vi "Fpga-Uart-State-Machine.vi"(6 "TX FIFO In":refnum<k21>="HT-UART_TX", 7 "RXD Pin In":refnum<k21>="UserRTL_d_microblaze_wrapper\\uart_rtl_rxd", 8 "RX FIFO In":refnum<k21>="TH-UART_RX", 9 "TXD Pin In":refnum<k21>="UserRTL_d_microblaze_wrapper\\uart_rtl_txd", 10 "Baud Rate":u32(ring)=128000 items=["110"=110, "300"=300, "1200"=1200, "2400"=2400, "4800"=4800, "9600"=9600, "19200"=19200, "38400"=38400, "57600"=57600, "115200"=115200, "128000"=128000, "230400"=230400, "460800"=460800, "921600"=921600], 11 "FPGA Clock Rate (MHz)":u32=100) -> ()   [LabVIEW 2018]
uses:
  <vilib>/Platform/TimedLoop/XDataNode/timing_clust.ctl
  <vilib>/Platform/TimedLoop/XDataNode/nitl_modes.ctl
  <vilib>/Platform/TimedLoop/XDataNode/wakeup.ctl
  UART.RX.States.2.ctl
  UART.RX.States.ctl
  <vilib>/rvi/Emulation/niFpgaSctlEmulationGetInTimedLoop.vi
  <vilib>/rvi/Emulation/niFpgaEmulationReportErrorSimple.vi
  <vilib>/rvi/Emulation/niFpgaGetClockAttributes.vi
  <vilib>/rvi/Emulation/niFpgaCriticalErrorInLSC.vi
  <vilib>/rvi/eio/common/nirviEmuTemplateMethod_errors.vi
  <vilib>/rvi/DataTransferAndStorage/Container/Common/niFpgaContainerExecOnDevCompGetState.vi
  <vilib>/rvi/Emulation/niFpgaEmulationIsFPGAContextNoSignature.vi
  <vilib>/rvi/errors/niFpgaSetErrorForExecOnDevCompSimple.vi
  <vilib>/rvi/eio/common/nirviEmuReportErrorAndStop.vi
  <vilib>/rvi/DataTransferAndStorage/Container/Common/niFpgaContainerGetUniqueNameForEmu.vi
  <vilib>/rvi/FIFO/Fifo_Resource/nirvififoEmulationSetSize.vi
  <vilib>/rvi/FIFO/Fifo_Resource/nirviFifoEmulationQueueMgr.vi
  <instcachedir>/0/nirviFifoEmulationQueueMgr_E5CAEC123FF24DC58D834DCA3CDAA9B5.lvgen/nirviFifoEmulationQueueMgr_E5CAEC123FF24DC58D834DCA3CDAA9B5_001.vi
  <vilib>/rvi/FIFO/Fifo_Resource/nirvififoEmulationDetermineInputValidOut.vi
  <vilib>/rvi/FIFO/Fifo_Resource/nirvififoEmulationCreateLock.vi
  <vilib>/rvi/Emulation/niFpgaProcessEmulError.vi
  <vilib>/rvi/FIFO/Fifo_Resource/nirvififoEmulationObtainLock.vi
  <vilib>/rvi/FIFO/Fifo_Resource/nirvififoEmulationReleaseLock.vi
  <vilib>/rvi/occurrence/nirviWaitOnOccurrenceBase.vi
  <vilib>/rvi/errors/nirviReportUnexpectedCaseInternalError.vi
  <vilib>/rvi/errors/nirviReportUnexpectedCaseInternalError (U32).vi
  <vilib>/Utility/error.llb/Clear Errors.vi
  <vilib>/rvi/interface/RandomDataEmulation/niFpgaRandomDataHandleErrors.vi
  <vilib>/Platform/TimedLoop/XDataNode/XDataNode.xnode
  <vilib>/eio/EIONode/EIONode.xnode
  <vilib>/rvi/DataTransferAndStorage/Container/XNode/niFpgaContainer.xnode
  <vilib>/rvi/FIFO/Fifo_Resource/niFpgaFifoEmulationRefIn.vi
  <vilib>/Platform/TimedLoop/XDataNode/XDNodeRunTimeDep.lvlib
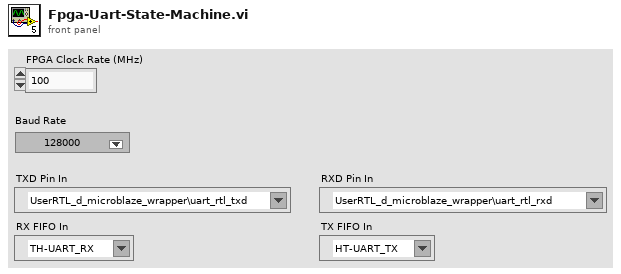
[diagram p1: front panel]
types:
  T1 = typedef "XDNodeRunTimeDep.lvlib/timing_clust.ctl" = cluster{"Expected End [f-1]":u64, "Actual End [f-1]":u64, "Finished Late? [f-1]":bool, "Expected End [i-1]":u64, "Actual End [i-1]":u64, "Finished Late? [i-1]":bool, "Expected Start [i]":u64, "Actual Start [i]":u64, "Expected Start [f]":u64, "Actual Start [f]":u64, "Source Name":string, "Structure Name":string, "Period":i64, "Deadline":i64, "Offset":i64, "Start":i64, "Priority":i32, "Timeout":i32, "Mode":T2, "Wakeup Reason":T3, "Error":errorcluster, "Source Type":string, "Secondary Source Type":string, "Global End Time":u64, "Global Start Time":u64, "Frame Duration":u64, "Iteration Duration":u64, "Assigned CPU":i32, "I/O Scan Engine Mode":u32}
  T2 = typedef "XDNodeRunTimeDep.lvlib/nitl_modes.ctl" = enum32{"No Change", "Process missed periods, maintain original phase", "Discard missed periods, maintain original phase", "Process missed periods, ignore original phase", "Discard missed periods, ignore original phase"}
  T3 = typedef "XDNodeRunTimeDep.lvlib/wakeup.ctl" = enum32{"Normal", "Aborted", "Asynchronous wakeup", "Timing source error", "Timed loop error", "Timeout"}
  T4 = typedef "UART.RX.States.2.ctl" = enum16{"No-Wait", "Wait-Half", "Wait-Full", "Wait-One-and-a-Half"}
  T5 = typedef "UART.RX.States.ctl" = enum16{"Read-StartBit", "Read-DataBits", "Read-Parity", "Read-StopBit", "Shift"}
  T6 = enum16{"Wait.for.New", "Send.StartBit", "Send.DataBits", "Send.Parity", "Send.StopBit"}
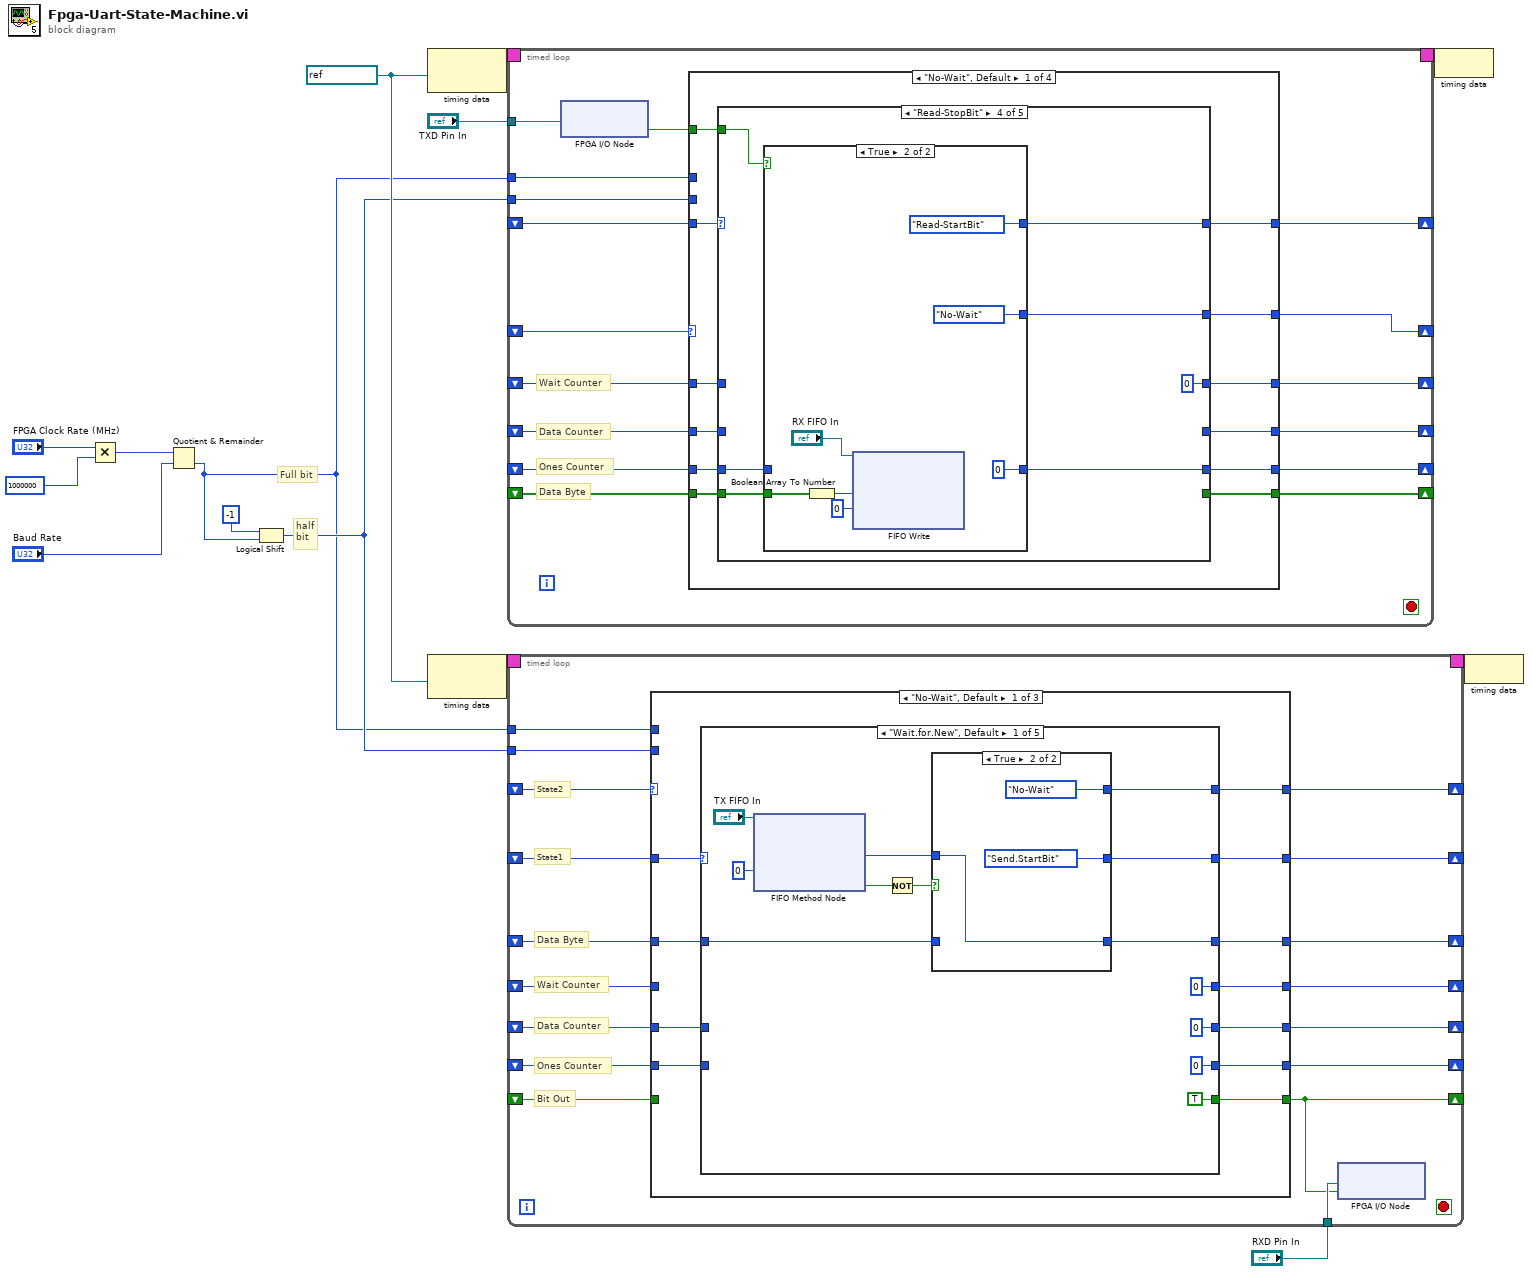
[diagram p0: block diagram]
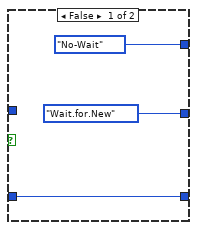
[diagram p2: hidden frame]
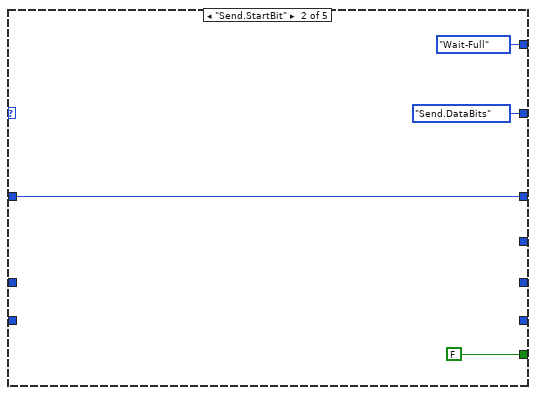
[diagram p3: hidden frame]
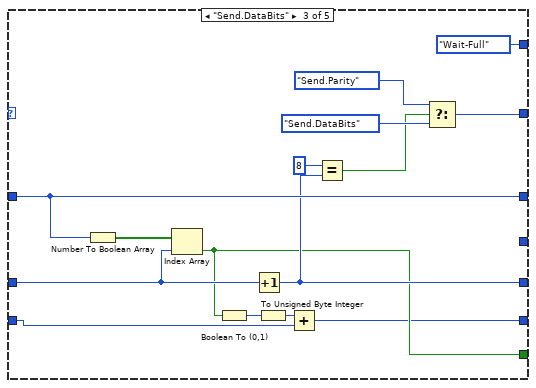
[diagram p4: hidden frame]
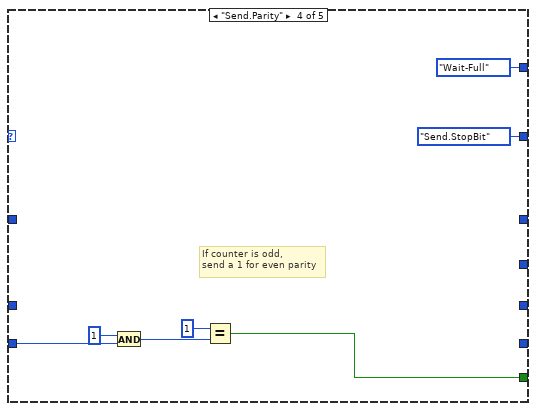
[diagram p5: hidden frame]
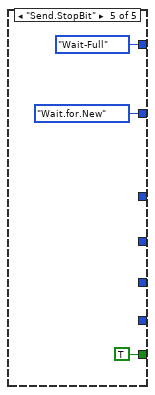
[diagram p6: hidden frame]
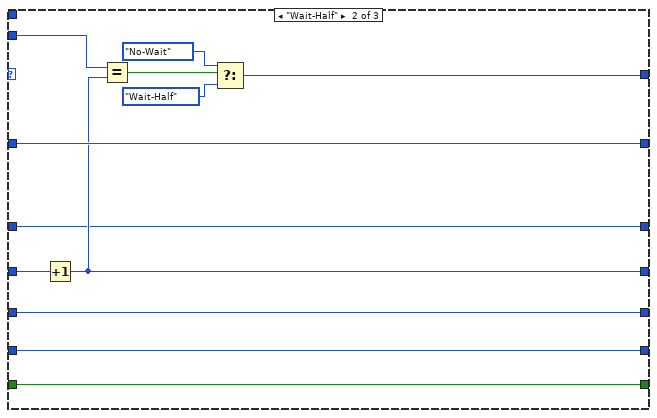
[diagram p7: hidden frame]
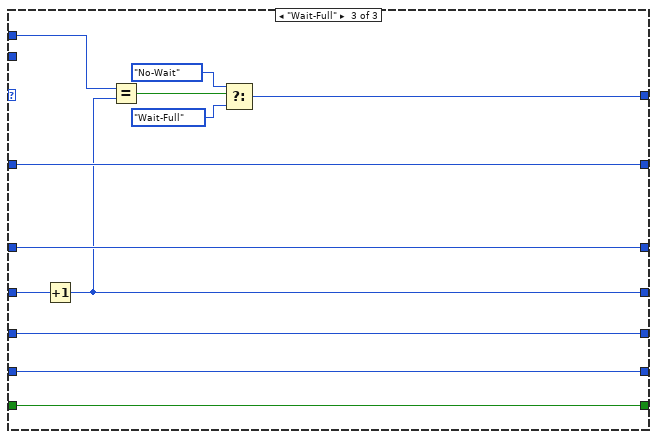
[diagram p8: hidden frame]
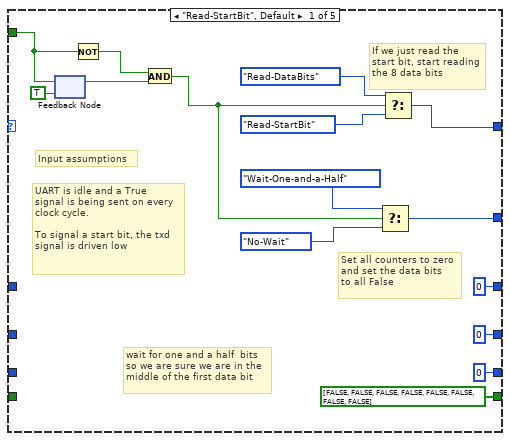
[diagram p9: hidden frame]
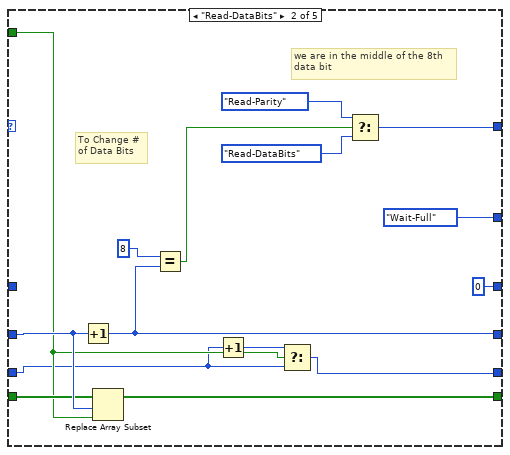
[diagram p10: hidden frame]
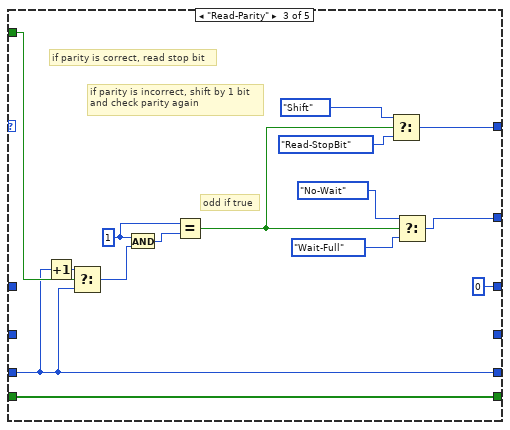
[diagram p11: hidden frame]
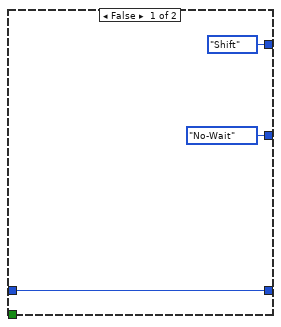
[diagram p12: hidden frame]
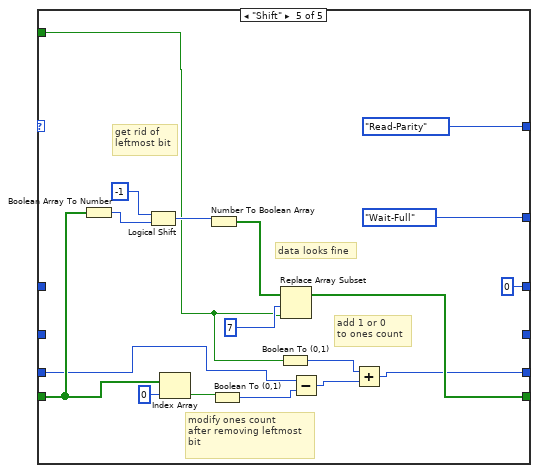
[diagram p13: hidden frame]
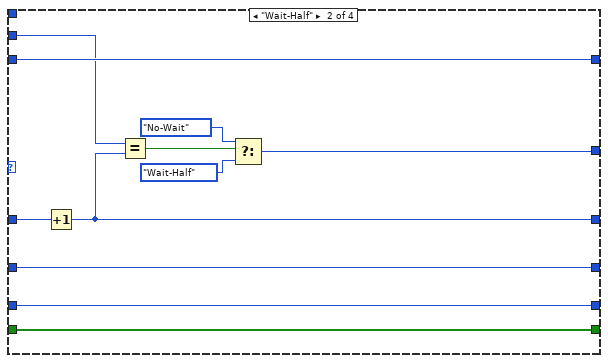
[diagram p14: hidden frame]
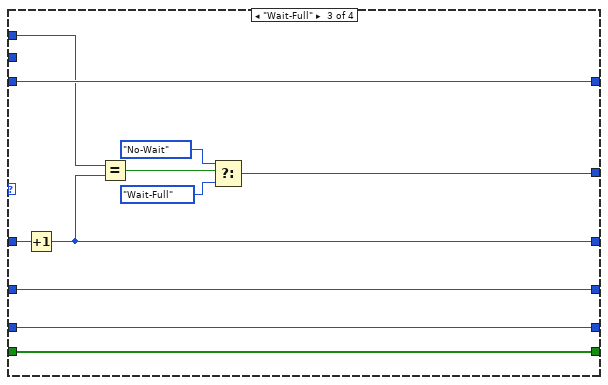
[diagram p15: hidden frame]
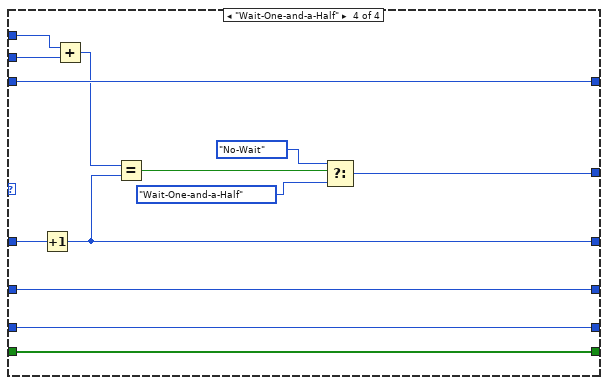
[diagram p16: hidden frame]
diagram:
  w3 = refnum<k21> "100MHz" ("Source Name")
  # "half\nbit"
  # "Full bit"
  n1 = Multiply(x="FPGA Clock Rate (MHz)", y=u32 1000000) -> (x*y=w13:u32)
  n2 = Quotient & Remainder(x=w13, y="Baud Rate") -> (floor(x/y)=w1:u32)  [unwired: 1 out]
  n3 = Logical Shift(y=i16 -1, x=w1) -> (x << y=w2:u32)
  n4 = node-c288(w3) -> (w10:T1)
  n5 = node-c288(w3) -> (w6:T1)
  n6 = timed-loop {
    timing: w10 -> [_]
    timing-out: [_] -> w9
    shift-right: [w29] -> _
    shift-left: _ -> [w30]
    shift-right: [w27] -> _
    shift-left: _ -> [w28]
    shift-right: [w24] -> _
    shift-left: _ -> [w26]
    shift-right: [w23] -> _
    shift-left: _ -> [w25]
    tunnel: w1 -> [w22]
    tunnel: w2 -> [w21]
    shift-right: [w20] -> _
    shift-left: _ -> [w19]
    shift-right: [w17] -> _
    shift-left: _ -> [w18]
    tunnel: "TXD Pin In" -> [w16]
    stop <- _ stop-if-true
    # "Data Byte"
    # "Ones Counter"
    # "Data Counter"
    # "Wait Counter"
    n7 = xnode "FPGA I/O Node"("FPGA I/O In"=w16) -> ("I/O Item"=w15:bool)  [unwired: 1 out]
    n8 = case shown="\"No-Wait\", Default" w28 {
      tunnel: w30 -> [w38 w127 w136 w149]
      tunnel: w15 -> [w31 _ _ _]
      tunnel: [w37 w127 w136 w149] -> w29
      tunnel: [w36 w128 w140 w153] -> w27
      tunnel: w26 -> [w42 w133 w141 w154]
      tunnel: w25 -> [w41 w126 w139 w152]
      tunnel: [w35 w132 w138 w151] -> w24
      tunnel: [w34 w126 w139 w152] -> w23
      tunnel: w22 -> [_ _ w135 w147]
      tunnel: w21 -> [_ w124 _ w146]
      tunnel: [w32 w125 w137 w150] -> w20
      tunnel: w19 -> [w40 w125 w137 w150]
      tunnel: w18 -> [w39 w123 w134 w148]
      tunnel: [w33 w123 w134 w148] -> w17
      frame "No-Wait", Default {
        n9 = case shown="\"Read-StopBit\"" w38 {
          tunnel: w31 -> [w54 w62 w87 w93 w109]
          tunnel: [w53 w63 w83 w91 UART.RX.States."Read-Parity"] -> w37
          tunnel: [w47 UART.RX.States.2."Wait-Full" w78 w92 UART.RX.States.2."Wait-Full"] -> w36
          tunnel: w42 -> [_ _ _ _ _]
          tunnel: w41 -> [_ w71 _ _ _]
          tunnel: [u32 0 ("Wait Counter") u32 0 ("Wait Counter") u32 0 ("Wait Counter") u32 0 ("Wait Counter") u32 0 ("Wait Counter")] -> w35
          tunnel: [u32 0 ("Data Counter") w68 _ _ _] -> w34
          tunnel: [bool[] [FALSE, FALSE, FALSE, FALSE, FALSE, FALSE, FALSE, FALSE] w69 w76 _ w115] -> w32
          tunnel: w40 -> [_ w70 w76 w94 w114]
          tunnel: w39 -> [_ w61 w74 w89 w112]
          tunnel: [u32 0 ("Data Counter") w59 w74 w90 w107] -> w33
          frame "Read-StartBit", Default {
            # "Set all counters to zero\nand set the data bits\nto all False"
            # "wait for one and a half  bits\nso we are sure we are in the\nmiddle of the first data bit"
            # "If we just read the \nstart bit, start reading\nthe 8 data bits"
            # "UART is idle and a True\nsignal is being sent on every\nclock cycle.\n\nTo signal a start bit, the txd\nsignal is driven low"
            # "Input assumptions"
            n10 = feedback #1(TRUE ("d_microblaze_i\\uart_rtl_txd")) -> (w57:bool)
            n11 = feedback-in #1(w54) -> ()
            n12 = Not(x=w54) -> (.not. x?=w56:bool)
            n13 = And(x=w56, y=w57) -> (x .and. y?=w50:bool)
            n14 = Select(t=UART.RX.States.2."Wait-One-and-a-Half", s=w50, f=UART.RX.States.2."No-Wait") -> (s? t:f=w47:T4)
            n15 = Select(t=UART.RX.States."Read-DataBits", s=w50, f=UART.RX.States."Read-StartBit") -> (s? t:f=w53:T5)
          }
          frame "Read-DataBits" {
            # "we are in the middle of the 8th\ndata bit"
            # "To Change #\nof Data Bits"
            n16 = Increment(x=w71) -> (x+1=w68:u32)
            n17 = Replace Array Subset(array=w70, new element=w62, index=w71) -> (w69:bool[])
            n18 = Equal?(x=u32 8, y=w68) -> (x = y?=w66:bool)
            n19 = Increment(x=w61) -> (x+1=w60:u32)
            n20 = Select(t=w60, s=w62, f=w61) -> (s? t:f=w59:u32)
            n21 = Select(t=UART.RX.States."Read-Parity", s=w66, f=UART.RX.States."Read-DataBits") -> (s? t:f=w63:T5)
          }
          frame "Read-Parity" {
            w84 = u32 1 ("x")
            # "odd if true"
            # "if parity is incorrect, shift by 1 bit\nand check parity again"
            # "if parity is correct, read stop bit"
            n22 = Increment(x=w74) -> (x+1=w86:u32)
            n23 = Select(t=w86, s=w87, f=w74) -> (s? t:f=w75:u32)
            n24 = And(x=w84, y=w75) -> (x .and. y?=w85:u32)
            n25 = Equal?(x=w84, y=w85) -> (x = y?=w80:bool)
            n26 = Select(t=UART.RX.States."Shift", s=w80, f=UART.RX.States."Read-StopBit") -> (s? t:f=w83:T5)
            n27 = Select(t=UART.RX.States.2."No-Wait", s=w80, f=UART.RX.States.2."Wait-Full") -> (s? t:f=w78:T4)
          }
          frame "Read-StopBit" {
            n28 = case shown="True" w93 {
              tunnel: w94 -> [_ w102]
              tunnel: [UART.RX.States.2."No-Wait" UART.RX.States.2."No-Wait"] -> w92
              tunnel: [UART.RX.States."Shift" UART.RX.States."Read-StartBit"] -> w91
              tunnel: [w95 u32 0 ("Ones Counter")] -> w90
              tunnel: w89 -> [w95 _]
              frame False {
              }
              frame True {
                n29 = Boolean Array To Number(Boolean array=w102) -> (number=w104:u8)
                n30 = xnode ("FIFO Write")("Element"=w104, "Timeout"=0, "FIFO In"="RX FIFO In") -> ()  [unwired: 2 out]
              }
            }
          }
          frame "Shift" {
            # "data looks fine"
            # "add 1 or 0\nto ones count"
            # "modify ones count\nafter removing leftmost\nbit"
            # "get rid of\nleftmost bit"
            n31 = Boolean Array To Number(Boolean array=w114) -> (number=w122:u8)
            n32 = Logical Shift(y=i16 -1, x=w122) -> (x << y=w120:u8)
            n33 = Index Array(array=w114, index=0) -> (element=w113:bool)
            n34 = Number To Boolean Array(number=w120) -> (Boolean array=w117:bool[])
            n35 = Boolean To (0,1)(Boolean=w113) -> (0, 1=w111:i16)
            n36 = Boolean To (0,1)(Boolean=w109) -> (0, 1=w108:i16)
            n37 = Replace Array Subset(array=w117, new element=w109, index=7) -> (w115:bool[])
            n38 = Subtract(x=w112, y=w111) -> (x-y=w110:u32)
            n39 = Add(x=w108, y=w110) -> (x+y=w107:u32)
          }
        }
      }
      frame "Wait-Half" {
        n40 = Increment(x=w133) -> (x+1=w132:u32)
        n41 = Equal?(x=w124, y=w132) -> (x = y?=w131:bool)
        n42 = Select(t=UART.RX.States.2."No-Wait", s=w131, f=UART.RX.States.2."Wait-Half") -> (s? t:f=w128:T4)
      }
      frame "Wait-Full" {
        n43 = Increment(x=w141) -> (x+1=w138:u32)
        n44 = Equal?(x=w135, y=w138) -> (x = y?=w144:bool)
        n45 = Select(t=UART.RX.States.2."No-Wait", s=w144, f=UART.RX.States.2."Wait-Full") -> (s? t:f=w140:T4)
      }
      frame "Wait-One-and-a-Half" {
        n46 = Increment(x=w154) -> (x+1=w151:u32)
        n47 = Add(x=w147, y=w146) -> (x+y=w145:u32)
        n48 = Equal?(x=w145, y=w151) -> (x = y?=w157:bool)
        n49 = Select(t=UART.RX.States.2."No-Wait", s=w157, f=UART.RX.States.2."Wait-One-and-a-Half") -> (s? t:f=w153:T4)
      }
    }
  }
  n50 = timed-loop {
    timing: w6 -> [_]
    timing-out: [_] -> w5
    shift-right: [w171] -> _
    shift-left: _ -> [w175]
    shift-right: [w174] -> _
    shift-left: _ -> [w176]
    shift-right: [w173] -> _
    shift-left: _ -> [w172]
    shift-right: [w170] -> _
    shift-left: _ -> [w169]
    tunnel: w2 -> [w168]
    tunnel: w1 -> [w167]
    tunnel: "RXD Pin In" -> [w166]
    shift-right: [w165] -> _
    shift-left: _ -> [w164]
    shift-right: [w163] -> _
    shift-left: _ -> [w162]
    shift-right: [w161] -> _
    shift-left: _ -> [w160]
    stop <- _ stop-if-true
    # "Ones Counter"
    # "Bit Out"
    # "Data Counter"
    # "Data Byte"
    # "State1"
    # "State2"
    # "Wait Counter"
    n51 = case shown="\"No-Wait\", Default" w175 {
      tunnel: w176 -> [w187 w241 w253]
      tunnel: [w186 w241 w253] -> w174
      tunnel: [w185 w237 w251] -> w173
      tunnel: w172 -> [w184 w237 w251]
      tunnel: [w183 w244 w256] -> w171
      tunnel: [w182 w238 w250] -> w170
      tunnel: w169 -> [_ w243 w255]
      tunnel: w168 -> [_ w242 _]
      tunnel: w167 -> [_ _ w254]
      tunnel: [w181 w240 w252] -> w165
      tunnel: w164 -> [_ w240 w252]
      tunnel: [w180 w239 w249] -> w163
      tunnel: w162 -> [w179 w239 w249]
      tunnel: [w178 w236 w248] -> w161
      tunnel: w160 -> [w177 w236 w248]
      frame "No-Wait", Default {
        n52 = case shown="\"Wait.for.New\", Default" w187 {
          tunnel: [w196 T6."Send.DataBits" w218 T6."Send.StopBit" T6."Wait.for.New"] -> w186
          tunnel: [w194 w207 w223 _ _] -> w185
          tunnel: w184 -> [w192 w207 w223 _ _]
          tunnel: [w195 UART.RX.States.2."Wait-Full" UART.RX.States.2."Wait-Full" UART.RX.States.2."Wait-Full" UART.RX.States.2."Wait-Full"] -> w183
          tunnel: [u32 0 ("Wait Counter") _ _ _ _] -> w182
          tunnel: [TRUE ("I/O Item") FALSE ("I/O Item") w215 w226 TRUE ("I/O Item")] -> w181
          tunnel: [u8 0 ("Wait Counter") _ w221 _ _] -> w180
          tunnel: w179 -> [_ _ w224 _ _]
          tunnel: [u8 0 ("Wait Counter") _ w214 _ _] -> w178
          tunnel: w177 -> [_ _ w212 w230 _]
          frame "Wait.for.New", Default {
            n53 = xnode ("FIFO Method Node")("Timeout"=0, "FIFO In"="TX FIFO In") -> ("Element"=w193:u8, "Timed Out?"=w198:bool)  [unwired: 1 out]
            n54 = Not(x=w198) -> (.not. x?=w197:bool)
            n55 = case shown="True" w197 {
              tunnel: [T6."Wait.for.New" T6."Send.StartBit"] -> w196
              tunnel: [UART.RX.States.2."No-Wait" UART.RX.States.2."No-Wait"] -> w195
              tunnel: [w201 w204] -> w194
              tunnel: w193 -> [_ w204]
              tunnel: w192 -> [w201 _]
              frame False {
              }
              frame True {
              }
            }
          }
          frame "Send.StartBit" {
          }
          frame "Send.DataBits" {
            n56 = Number To Boolean Array(number=w223) -> (Boolean array=w225:bool[])
            n57 = Index Array(array=w225, index=w224) -> (element=w215:bool)
            n58 = Boolean To (0,1)(Boolean=w215) -> (0, 1=w213:i16)
            n59 = Increment(x=w224) -> (x+1=w221:u8)
            n60 = To Unsigned Byte Integer(number=w213) -> (unsigned 8bit integer=w211:u8)
            n61 = Add(x=w211, y=w212) -> (x+y=w214:u8)
            n62 = Equal?(x=u8 8, y=w221) -> (x = y?=w217:bool)
            n63 = Select(t=T6."Send.Parity", s=w217, f=T6."Send.DataBits") -> (s? t:f=w218:T6)
          }
          frame "Send.Parity" {
            # "If counter is odd,\nsend a 1 for even parity"
            n64 = And(x=i16 1, y=w230) -> (x .and. y?=w228:i16)
            n65 = Equal?(x=i16 1, y=w228) -> (x = y?=w226:bool)
          }
          frame "Send.StopBit" {
          }
        }
      }
      frame "Wait-Half" {
        n66 = Increment(x=w243) -> (x+1=w238:u32)
        n67 = Equal?(x=w242, y=w238) -> (x = y?=w247:bool)
        n68 = Select(t=UART.RX.States.2."No-Wait", s=w247, f=UART.RX.States.2."Wait-Half") -> (s? t:f=w244:T4)
      }
      frame "Wait-Full" {
        n69 = Increment(x=w255) -> (x+1=w250:u32)
        n70 = Equal?(x=w254, y=w250) -> (x = y?=w259:bool)
        n71 = Select(t=UART.RX.States.2."No-Wait", s=w259, f=UART.RX.States.2."Wait-Full") -> (s? t:f=w256:T4)
      }
    }
    n72 = xnode "FPGA I/O Node"("I/O Item"=w165, "FPGA I/O In"=w166) -> ()  [unwired: 1 out]
  }
  n73 = node-c288(w9) -> ()
  n74 = node-c288(w5) -> ()
